vi "test2.vi"() -> ()   [LabVIEW 2015]
panel:
  out "Qty":string[](array[string])
  out "Descr":string[](array[string])
  out "S/N":string[](array[string])
  out "P/N":string[](array[string])
  out "numInvoice":string
  out "numItems":string
  out "date":string
  out "text 2":string[](array[string])
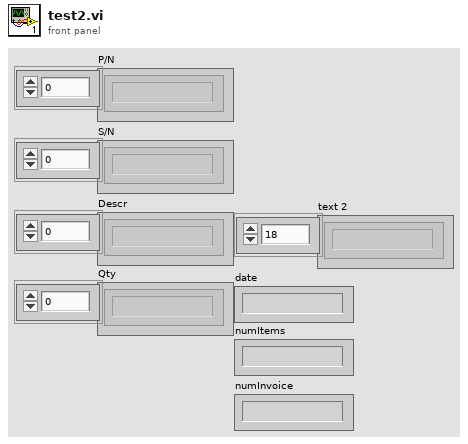
[diagram p1: front panel]
types:
  T1 = enum16{"date", "numItems", "numInvoice", "DataWithQty", "DataNoQty", "NextData", "Stop"}
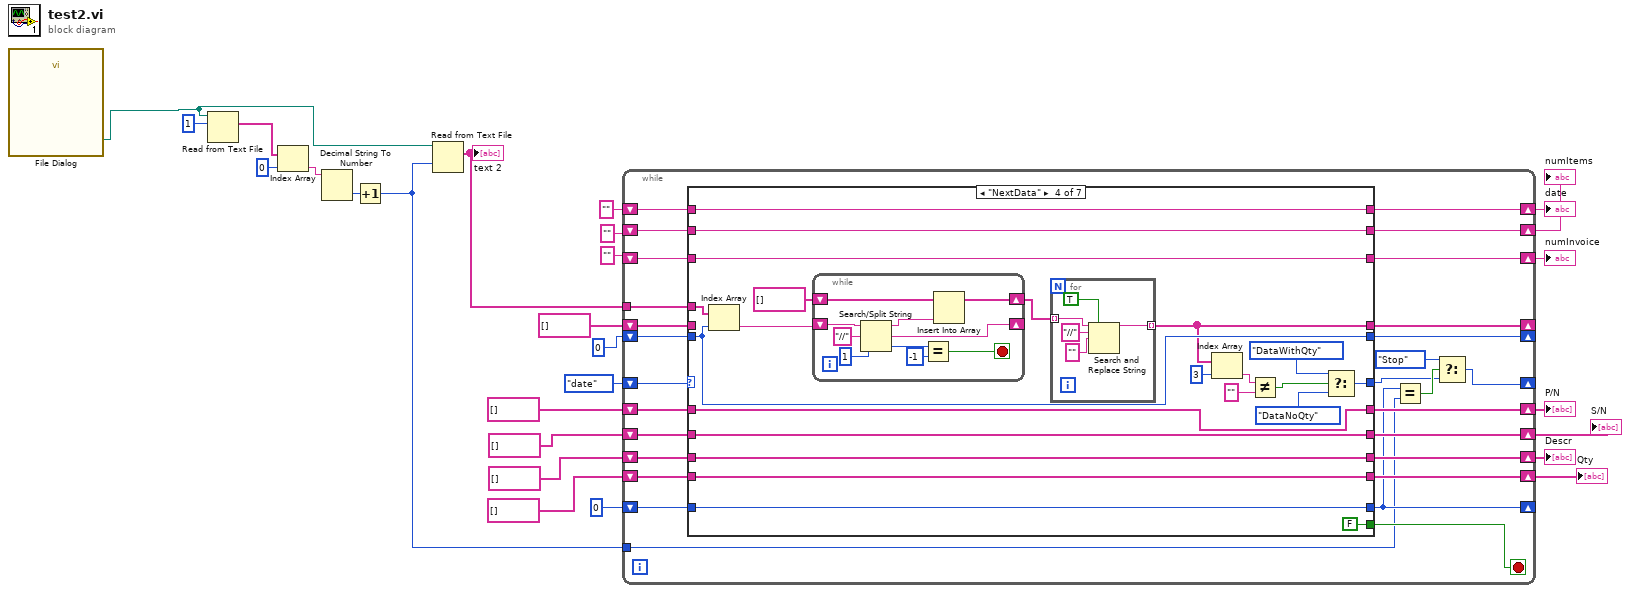
[diagram p0: block diagram]
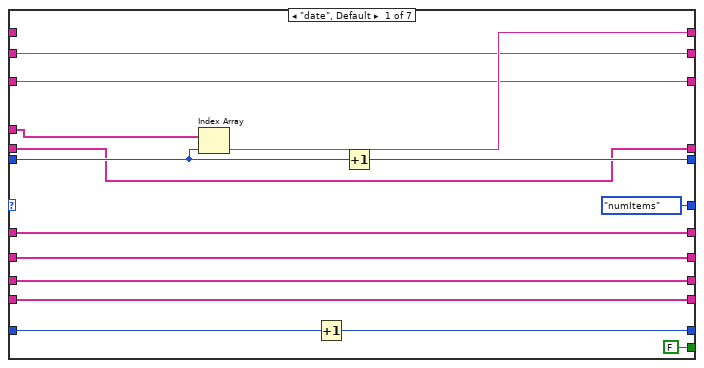
[diagram p2: hidden frame]
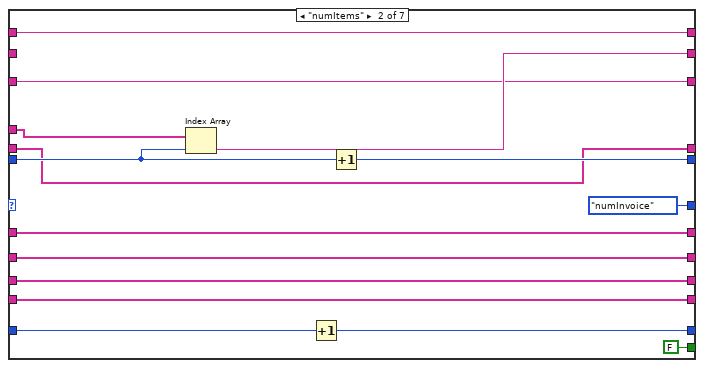
[diagram p3: hidden frame]
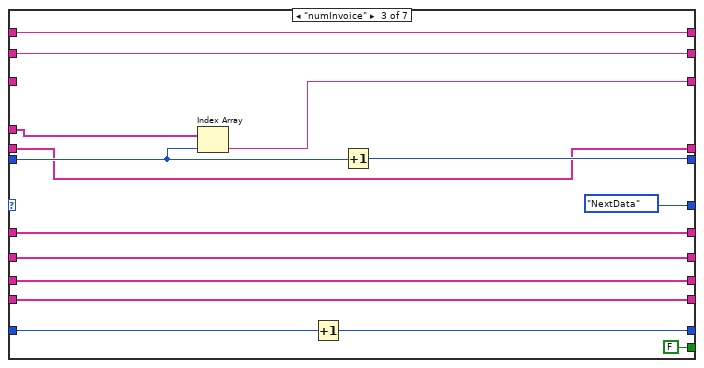
[diagram p4: hidden frame]
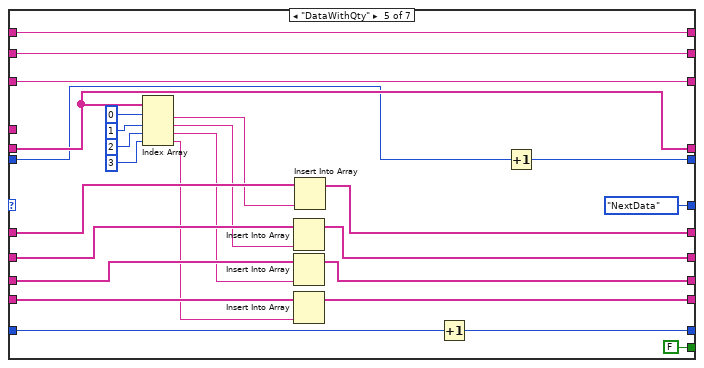
[diagram p5: hidden frame]
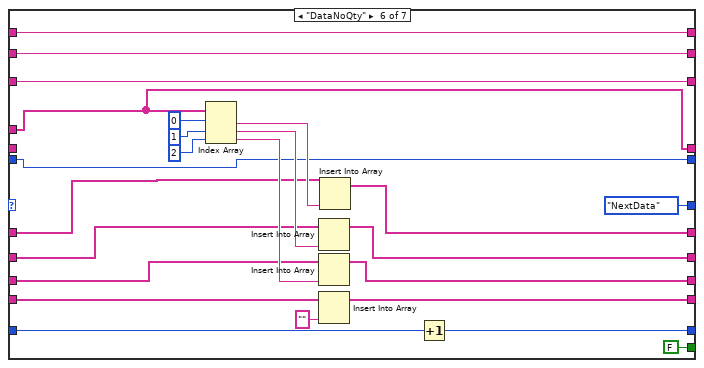
[diagram p6: hidden frame]
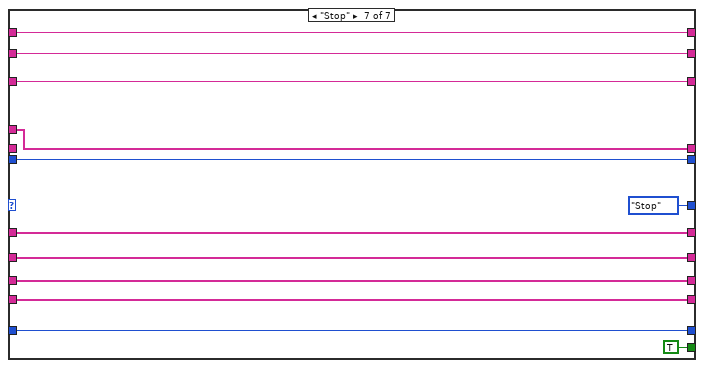
[diagram p7: hidden frame]
diagram:
  n1 = call "File Dialog"() -> ("selected path"=w1:path)  [unwired: 12 in, 3 out]
  n2 = Read from Text File(file (use dialog)=w1, count=1) -> (text=w6:string[])  [unwired: 2 in, 3 out]
  n3 = Index Array(array=w6, index=0) -> (element=w4:string)
  n4 = Decimal String To Number(string=w4) -> (number=w3:i32)  [unwired: 2 in, 1 out]
  n5 = Increment(x=w3) -> (x+1=w2:i32)
  n6 = Read from Text File(file (use dialog)=w1, count=w2) -> (text=w26:string[])  [unwired: 2 in, 3 out]
  "text 2" <- w26
  n7 = while {
    tunnel: w26 -> [w54]
    shift-right: [w28] -> _
    shift-left: T1."date" -> [w53]
    shift-right: [w50] -> _
    shift-left: 0 -> [w52]
    shift-right: [w51] -> w14
    shift-left: "" -> [w48]
    shift-right: [w49] -> w13
    shift-left: "" -> [w47]
    shift-right: [w46] -> w12
    shift-left: "" -> [w45]
    shift-right: [w44] -> _
    shift-left: string[] [] -> [w43]
    shift-right: [w32] -> _
    shift-left: 0 -> [w42]
    shift-right: [w37] -> w11
    shift-left: string[] [] -> [w41]
    shift-right: [w36] -> w10
    shift-left: string[] [] -> [w40]
    shift-right: [w35] -> w9
    shift-left: string[] [] -> [w39]
    shift-right: [w34] -> w8
    shift-left: string[] [] -> [w38]
    tunnel: w2 -> [w31]
    stop <- w33 stop-if-true
    n8 = case shown="\"NextData\"" w53 {
      tunnel: w54 -> [w69 w84 w98 w118 _ w167 w195]
      tunnel: w52 -> [w63 w83 w99 w114 w139 w166 w194]
      tunnel: [w68 w81 w97 w121 w162 w186 w198] -> w51
      tunnel: [w67 w79 w94 w114 w138 w166 w194] -> w50
      tunnel: [T1."numItems" T1."numInvoice" T1."NextData" w111 T1."NextData" T1."NextData" T1."Stop"] -> w29
      tunnel: [w65 w82 w96 w120 w161 w185 w197] -> w49
      tunnel: w48 -> [_ w81 w97 w121 w162 w186 w198]
      tunnel: w47 -> [w65 _ w96 w120 w161 w185 w197]
      tunnel: [w64 w78 w95 w119 w160 w184 w196] -> w46
      tunnel: w45 -> [w64 w78 _ w119 w160 w184 w196]
      tunnel: [w62 w77 w92 w113 w141 w167 w195] -> w44
      tunnel: w43 -> [w62 w77 w92 _ w141 _ _]
      tunnel: w42 -> [w61 w76 w91 w105 w159 w183 w187]
      tunnel: [w55 w70 w85 w105 w158 w163 w187] -> w32
      tunnel: w41 -> [w60 w75 w90 w104 w153 w176 w192]
      tunnel: w40 -> [w59 w74 w89 w103 w152 w175 w191]
      tunnel: w39 -> [w58 w73 w88 w102 w151 w174 w190]
      tunnel: w38 -> [w57 w72 w87 w101 w150 w173 w189]
      tunnel: [w60 w75 w90 w104 w145 w168 w192] -> w37
      tunnel: [w59 w74 w89 w103 w144 w169 w191] -> w36
      tunnel: [w58 w73 w88 w102 w143 w170 w190] -> w35
      tunnel: [w57 w72 w87 w101 w142 w171 w189] -> w34
      tunnel: [FALSE FALSE FALSE FALSE FALSE FALSE TRUE] -> w33
      frame "date", Default {
        n9 = Index Array(array=w69, index=w63) -> (element=w68:string)
        n10 = Increment(x=w61) -> (x+1=w55:i32)
        n11 = Increment(x=w63) -> (x+1=w67:i32)
      }
      frame "numItems" {
        n12 = Index Array(array=w84, index=w83) -> (element=w82:string)
        n13 = Increment(x=w76) -> (x+1=w70:i32)
        n14 = Increment(x=w83) -> (x+1=w79:i32)
      }
      frame "numInvoice" {
        n15 = Index Array(array=w98, index=w99) -> (element=w95:string)
        n16 = Increment(x=w91) -> (x+1=w85:i32)
        n17 = Increment(x=w99) -> (x+1=w94:i32)
      }
      frame "NextData" {
        n18 = Index Array(array=w118, index=w114) -> (element=w116:string)
        n19 = while {
          shift-right: [w135] -> w115
          shift-left: string[] [] -> [w136]
          shift-right: [w131] -> _
          shift-left: w116 -> [w134]
          stop <- w129 stop-if-true
          n20 = Search/Split String(string=w134, search string/char (-)="//", offset (0)=1) -> (substring before match=w133:string, match + rest of string=w131:string, offset of match=w130:i32)
          n21 = Equal?(x=w130, y=-1) -> (x = y?=w129:bool)
          n22 = Insert Into Array(array=w136, new element=w133) -> (w135:string[])  [unwired: 1 in]
        }
        n23 = for {
          tunnel: [w123] -> w113 mode=indexing
          tunnel: w115 -> [w122] mode=indexing
          n24 = Search and Replace String(replace all?=TRUE ("replace all? (F)"), input string=w122, search string="//", replace string="" ("replace string (\"\")")) -> (result string=w123:string)  [unwired: 4 in, 3 out]
        }
        n25 = Index Array(array=w113, index=3) -> (element=w110:string)
        n26 = Not Equal?(x=w110, y="") -> (x != y?=w108:bool)
        n27 = Select(t=T1."DataWithQty", s=w108, f=T1."DataNoQty") -> (s? t:f=w111:T1)
      }
      frame "DataWithQty" {
        n28 = Index Array(array=w141, index #1=0, index #2=1, index #3=2, index #4=3) -> (element #1=w149:string, element #2=w148:string, element #3=w147:string, element #4=w146:string)
        n29 = Insert Into Array(array=w152, new element=w148) -> (w144:string[])  [unwired: 1 in]
        n30 = Insert Into Array(array=w151, new element=w147) -> (w143:string[])  [unwired: 1 in]
        n31 = Insert Into Array(array=w150, new element=w146) -> (w142:string[])  [unwired: 1 in]
        n32 = Insert Into Array(array=w153, new element=w149) -> (w145:string[])  [unwired: 1 in]
        n33 = Increment(x=w159) -> (x+1=w158:i32)
        n34 = Increment(x=w139) -> (x+1=w138:i32)
      }
      frame "DataNoQty" {
        n35 = Index Array(array=w167, index #1=0, index #2=1, index #3=2) -> (element #1=w179:string, element #2=w178:string, element #3=w177:string)
        n36 = Insert Into Array(array=w175, new element=w178) -> (w169:string[])  [unwired: 1 in]
        n37 = Insert Into Array(array=w174, new element=w177) -> (w170:string[])  [unwired: 1 in]
        n38 = Insert Into Array(array=w173, new element="" ("new element/subarray")) -> (w171:string[])  [unwired: 1 in]
        n39 = Insert Into Array(array=w176, new element=w179) -> (w168:string[])  [unwired: 1 in]
        n40 = Increment(x=w183) -> (x+1=w163:i32)
      }
      frame "Stop" {
      }
    }
    n41 = Equal?(x=w32, y=w31) -> (x = y?=w30:bool)
    n42 = Select(t=T1."Stop", s=w30, f=w29) -> (s? t:f=w28:T1)
  }
  "date" <- w14
  "numItems" <- w13
  "numInvoice" <- w12
  "P/N" <- w11
  "S/N" <- w10
  "Descr" <- w9
  "Qty" <- w8
